vi "Festival Main.vi"() -> ()   [LabVIEW 2013]
doc: "This example shows how to debounce a digital signal acquired from a push button switch."
uses:
  Controls/Key Store Actions.ctl
  Controls/ATT M2X Streams.ctl
  <vilib>/myRIO/Common/Instrument Driver Framework/myRIO v1.0/UART/vis/myRIO v1.0 Close UART.vi
  <vilib>/LVH/i3 Twitter/SubVIs/Twitter Open - Embedded.vi
  <vilib>/myRIO/Common/Instrument Driver Framework/Utilities/vis/FPGA Ref Manager.vi
  <vilib>/myRIO/Common/Instrument Driver Framework/myRIO v1.0/myRIO v1.0 Reset FPGA.vi
  <vilib>/LVH/i3 Twitter/i3-twitter.lvlib
  <vilib>/myRIO/Instrument Drivers/Utilities/Utilities.lvlib
panel:
  in  "Send to Servers":bool=TRUE
  out "error out":errorcluster
  # "Overview: This example shows how to debounce a digital signal acquired from a push button switch.\nInstructions:\n1. Connect an external push button switch to DIO0 on connector A.\n2. Check the myRIO target IP Address in the project and make sure the target IP Address is correct.\n3. Run this VI.\n4. Depending on the quality of the push button switch, you may or may not see jitter."
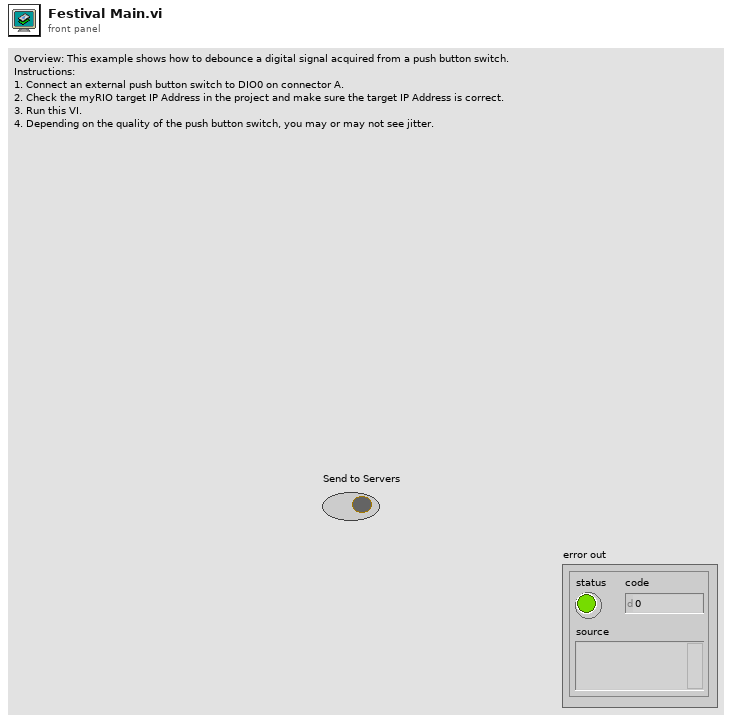
[diagram p1: front panel]
types:
  T1 = typedef "Key Store Actions.ctl" = enum16{"Load Keys File", "Get Keys", "Save Current Keys", "Save Manual Edit Keys"}
  T2 = typedef "ATT M2X Streams.ctl" = enum16{"tweets", "tweets-make"}
  T3 = typedef "JSON Key List.ctl" = cluster{"X-M2X-KEY":string, "M2X Feed ID":string, "Twitter Access Token":string, "Twitter Access Secret":string, "Twitter Client Token":string, "Twitter Client Secret":string, "NTP Server":string, "Beacons":cluster{"UUID":string, "Major":string, "Minor":string, "BT Address":string}[]}
  T4 = typedef "IMAQ Image.ctl" = refnum<image>
  T5 = typedef "i3-twitter.lvlib/Twitter Handle.ctl" = cluster{"OAuth Credentials":T6, "since ID":string, "max ID":string, "Screen Name":string}
  T6 = typedef "i3-oauth.lvlib/OAuth Handle.ctl" = cluster{"Signature Method":T7, "Version":string, "Client":T8, "Access":T8}
  T7 = typedef "i3-oauth.lvlib/Signature Method.ctl" = enum16{"HMAC-MD5", "HMAC-SHA1", "HMAC-SHA224", "HMAC-SHA256", "HMAC-SHA384", "HMAC-SHA512"}
  T8 = typedef "i3-oauth.lvlib/Credentials.ctl" = cluster{"Token":string, "Secret":string}
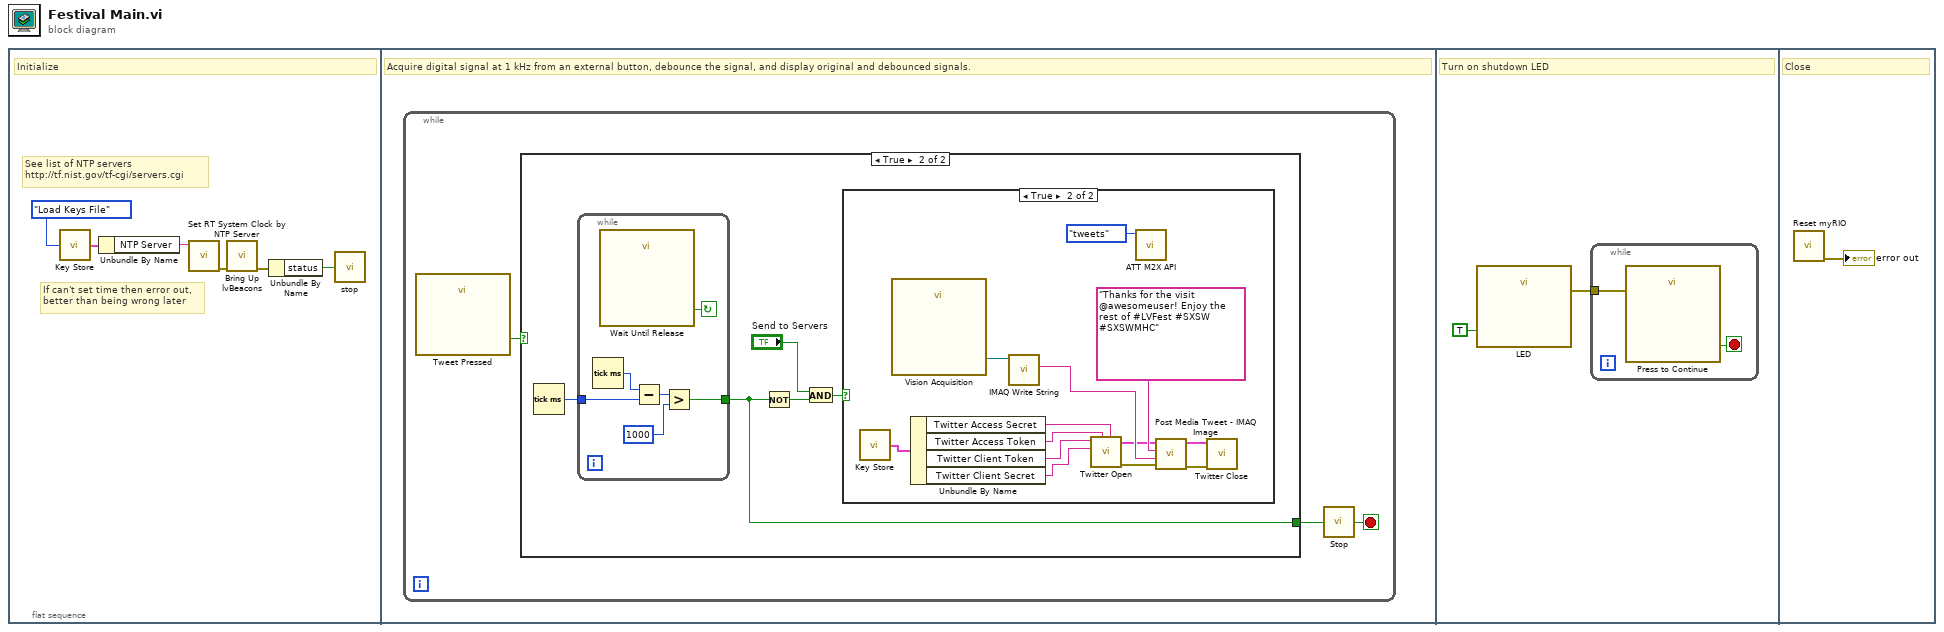
[diagram p0: block diagram]
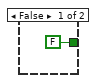
[diagram p2: hidden frame]
diagram:
  n1 = flat-sequence {
    frame #0 {
      # "If can't set time then error out,\nbetter than being wrong later"
      # "See list of NTP servers\nhttp://tf.nist.gov/tf-cgi/servers.cgi"
      # "Initialize"
      n2 = call "Key Store.vi"("Key Store Actions (default Get Keys)"=Key_Store_Actions."Load Keys File") -> ("Current Store"=w6:T3)
      n3 = Unbundle By Name(w6) -> ("NTP Server"=w5:string)
      n4 = call "Set RT System Clock by NTP Server.vi"("Time Server IP"=w5) -> ("error out"=w3:errorcluster)  [unwired: 9 in, 1 out]
      n5 = call "Bring Up lvBeacons.vi"("Error In"=w3) -> ("Error Out"=w2:errorcluster)  [unwired: 10 in]
      n6 = Unbundle By Name(w2) -> ("status"=w1:bool)
      n7 = call "stop.vi"("Stop?"=w1) -> ()  [unwired: 1 out]
    }
    frame #1 {
      # "Acquire digital signal at 1 kHz from an external button, debounce the signal, and display original and debounced signals."
      n8 = while {
        stop <- w8 stop-if-true
        n9 = call "Tweet Pressed"() -> ("Value"=w9:bool)  [unwired: 26 in, 1 out]
        n10 = case shown="True" w9 {
          tunnel: [FALSE w12] -> w7
          frame False {
          }
          frame True {
            n11 = Tick Count (ms)() -> (millisecond timer value=w11:u32)
            n12 = while {
              tunnel: [w31] -> w12
              tunnel: w11 -> [w30]
              stop <- w34 continue-if-true
              n13 = Tick Count (ms)() -> (millisecond timer value=w29:u32)
              n14 = call "Wait Until Release"() -> ("Value"=w34:bool)  [unwired: 26 in, 1 out]
              n15 = Subtract(x=w29, y=w30) -> (x-y=w33:u32)
              n16 = Greater?(x=w33, y=u32 1000) -> (0:w31:bool)
            }
            n17 = Not(x=w12) -> (.not. x?=w15:bool)
            n18 = And(x="Send to Servers", y=w15) -> (x .and. y?=w14:bool)
            n19 = case shown="True" w14 {
              frame False {
              }
              frame True {
                n20 = call "Key Store.vi"() -> ("Current Store"=w21:T3)  [unwired: 1 in]
                n21 = call "Vision Acquisition"() -> ("Image Out"=w25:T4)  [unwired: 1 in, 26 out]
                n22 = Unbundle By Name(w21) -> ("Twitter Access Secret"=w19:string, "Twitter Access Token"=w20:string, "Twitter Client Token"=w18:string, "Twitter Client Secret"=w17:string)
                n23 = call-poly "IMAQ Write String"("Image"=w25) -> ("FileString"=w24:string)  [unwired: 8 in, 2 out]
                n24 = call-poly <vilib>:"Twitter Open.vi"("Access Secret"=w19, "Access Token"=w20, "Consumer Secret"=w17, "Consumer Key"=w18) -> ("error out"=w23:errorcluster, "Twitter Handle Out"=w22:T5)  [unwired: 6 in]
                n25 = call "ATT M2X API.vi"("M2X Action"=ATT_M2X_Streams."tweets") -> ()  [unwired: 11 in]
                n26 = call "Post Media Tweet - IMAQ Image.vi"("error in"=w23, "PNG String"=w24, "Tweet"="Thanks for the visit @awesomeuser! Enjoy the rest of #LVFest #SXSW #SXSWMHC", "Twitter Handle In"=w22) -> ("error out"=w27:errorcluster, "Twitter Handle Out"=w26:T5)  [unwired: 6 in]
                n27 = call <vilib>:"Twitter Close.vi"("error in"=w27, "Twitter Handle In"=w26) -> ()  [unwired: 9 in, 1 out]
              }
            }
          }
        }
        n28 = call "Stop.vi"("Stop?"=w7) -> ("Stop Called"=w8:bool)
      }
    }
    frame #2 {
      # "Turn on shutdown LED"
      n29 = call "LED"("Shutdown"=TRUE) -> ("error out"=w35:errorcluster)  [unwired: 26 in]
      n30 = while {
        tunnel: w35 -> [w38]
        stop <- w37 stop-if-true
        n31 = call "Press to Continue"("error in (no error)"=w38) -> ("Value"=w37:bool)  [unwired: 25 in, 1 out]
      }
    }
    frame #3 {
      # "Close"
      n32 = call <vilib>:"Reset myRIO.vi"() -> ("error out"=→"error out":errorcluster)  [unwired: 11 in]
    }
  }
